vi "Intake Controller.vi"(8 "error in":errorcluster) -> ()   [LabVIEW 2017]
doc: "This VI executes continuously carrying out the current operation and responding to updates or new operations. It will often contain the timing or control code that is difficult to place directly in TeleOp. This VI generally opens all sensors and motors and isolates the rest of the robot code from knowing how the operations are carried out."
uses:
  Intake Operations.ctl
  Intake Setpoints.ctl
  <vilib>/Rock Robotics/WPI/SafetyOutput/WPI_SafetyOutputConfigMenu.ctl
  <vilib>/Rock Robotics/SystemInterfaces/DIO/FPGA_DIOPWMChannel.ctl
  <vilib>/Rock Robotics/WPI/RobotDrive/WPI_RobotDriveOpen2MotorWithSPARK.vi
  <vilib>/Rock Robotics/WPI/RobotDrive/WPI_RobotDriveOpen4MotorWithSPARK.vi
  <vilib>/Rock Robotics/Network Tables/NT Write Boolean.vi
  <vilib>/Rock Robotics/WPI/Solenoid/WPI_SolenoidOpenSingle.vi
  <vilib>/Rock Robotics/WPI/Solenoid/WPI_SolenoidChannel.ctl
  <vilib>/Rock Robotics/WPI/Framework/Completion Status.ctl
panel:
  in  "Interactive Values":T1
  out "Current\nCmd":string
  in  "Buttons":cluster{"Execute Cmd":bool, "Abort Cmd":bool}
  out "Command Timing":cluster{"Start Time (ms)":u32, "Iterations":i32}
  out "Status":T3
  # "Tip: It may be helpful to observe inputs and sensor values.\nYou may also want to display tuning or debugging controls."
  # "Interactive Command: You may fill in the settings for a command\nand schedule it with the Execute button. You can observe and abort\nany command while fine tuning the code for the controller."
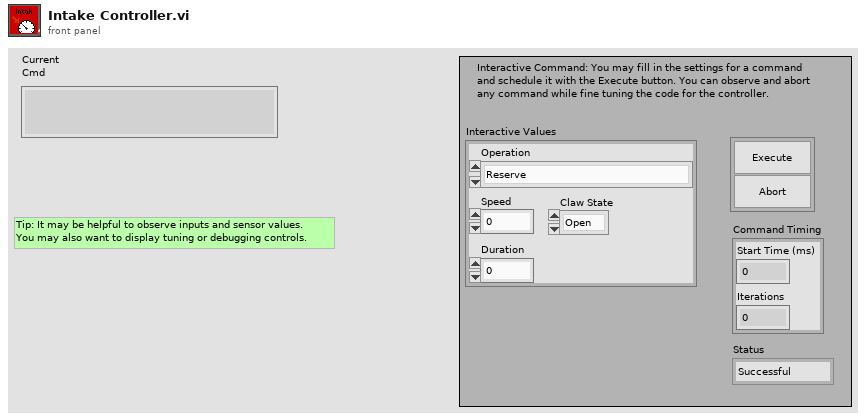
[diagram p1: front panel]
types:
  T1 = typedef "Intake Setpoints.ctl" = cluster{"Operation":T2, "Speed":dbl, "Duration":dbl, "Claw State":enum16{"Open", "Closed"}}
  T2 = typedef "Intake Operations.ctl" = enum16{"Reserve", "Read Current", "Immediate", "Open and Close Claw", "Intake for Duration", "Intake Until Cube"}
  T3 = typedef "Completion Status.ctl" = enum16{"Successful", "Aborted", "Incomplete"}
  T4 = typedef "WPI_SolenoidChannel.ctl" = enum8{"Solenoid 0", "Solenoid 1", "Solenoid 2", "Solenoid 3", "Solenoid 4", "Solenoid 5", "Solenoid 6", "Solenoid 7", "Invalid"}
  T5 = typedef "WPI_SafetyOutputConfigMenu.ctl" = enum16{"Enable", "Disable"}
  T6 = typedef "FPGA_DIOPWMChannel.ctl" = enum8{"PWM 0", "PWM 1", "PWM 2", "PWM 3", "PWM 4", "PWM 5", "PWM 6", "PWM 7", "PWM 8", "PWM 9", "PWM MXP 0", "PWM MXP 1", "PWM MXP 2", "PWM MXP 3", "PWM MXP 4", "PWM MXP 5", "PWM MXP 6", "PWM MXP 7", "PWM MXP 8", "PWM MXP 9", "Invalid"}
  T7 = typedef "WPI_RobotDriveDevRef.ctl" = cluster{"DevStatus":errorcluster, "Motors[]":T8[], "Square Inputs":bool, "Max Output":dbl}
  T8 = typedef "WPI_MotorControlDeviceRef.ctl" = cluster{"DeviceStatus":errorcluster, "Type":T9, "PWM":cluster{"PWM Channel":T6, "DeadBand":T10}, "CAN":cluster{"Device Number":u8, "SetOutput VI Ref":variant, "GetOutput VI Ref":variant, "Enable VI Ref":variant, "Disable VI Ref":variant, "Data":variant}, "Invert":bool, "DIO PWM":cluster{"PWM \"Enable\" Channel":T6, "DIOChannel":T11, "PWM Rate":dbl}}
  T9 = typedef "WPI_MotorControlType.ctl" = enum16{"PWM", "CAN", "DIO PWM"}
  T10 = typedef "WPI_PWMDeadband.ctl" = cluster{"Name":string, "maxPositivePwm":i32, "minPositivePwm":i32, "centerPwm":i32, "maxNegativePwm":i32, "minNegativePwm":i32, "angularRange":u16}
  T11 = typedef "FPGA_DIOChannel.ctl" = enum8{"DIO 0", "DIO 1", "DIO 2", "DIO 3", "DIO 4", "DIO 5", "DIO 6", "DIO 7", "DIO 8", "DIO 9", "DIO MXP 0", "DIO MXP 1", "DIO MXP 2", "DIO MXP 3", "DIO MXP 4", "DIO MXP 5", "DIO MXP 6", "DIO MXP 7", "DIO MXP 8", "DIO MXP 9", "DIO MXP 10", "DIO MXP 11", "DIO MXP 12", "DIO MXP 13", "DIO MXP 14", "DIO MXP 15", "SPI Port CS1", "SPI Port CS2", "SPI Port CS3", "SPI Port MISO", "SPI Port MOSI", "Invalid"}
  T12 = cluster{"RobotDriveDevRef":T7, "RobotDriveDevRef":T7}
  T13 = typedef "Command Status Info.ctl" = cluster{"Name":string, "Status":T3, "notifier out":T14}
  T14 = typedef "Completion Notifier.ctl" = refnum<notifier>
  T15 = cluster{"Current Command":T1, "Command Timing":cluster{"Start Time (ms)":u32, "Iterations":i32}, "Command Arguments":cluster{"Command Info":T13, "Description":string, "Default Command":T1, "queue out":refnum<queue>, "Subsystem Name":string}}
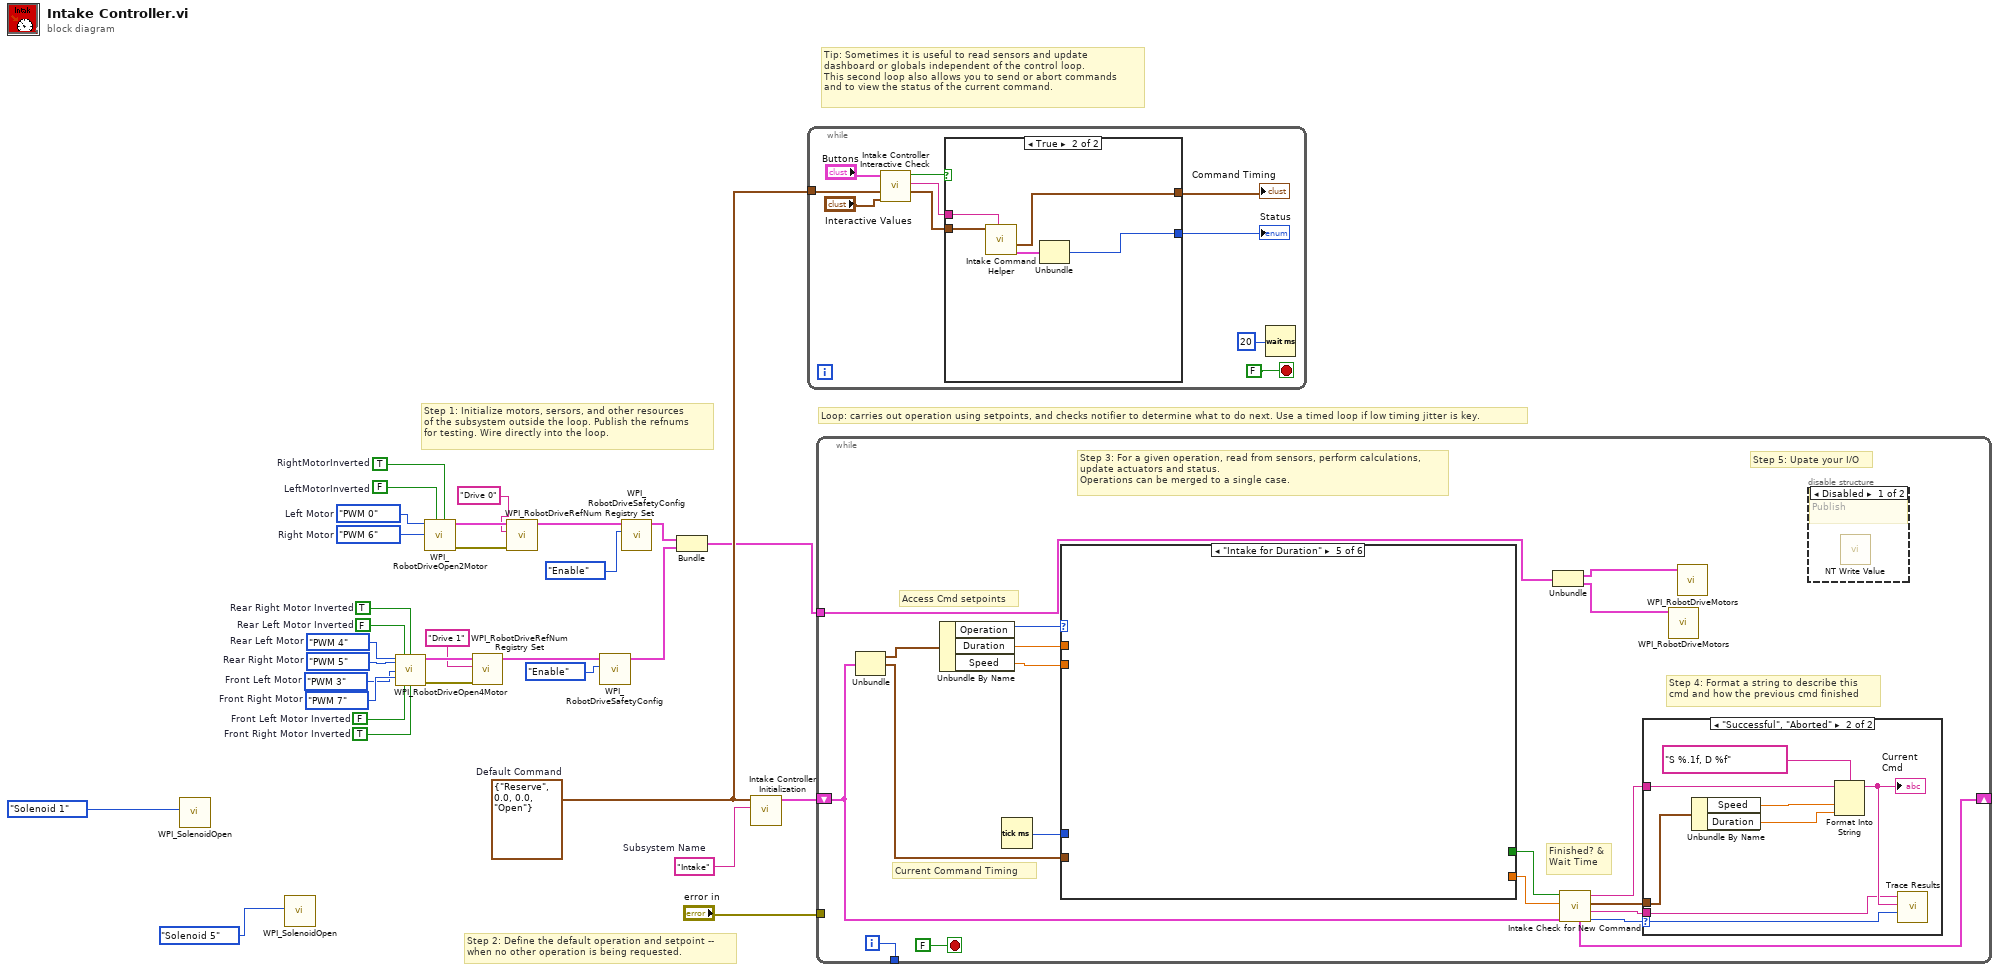
[diagram p0: block diagram]
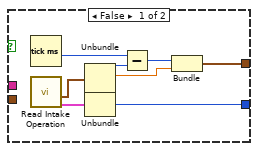
[diagram p2: hidden frame]
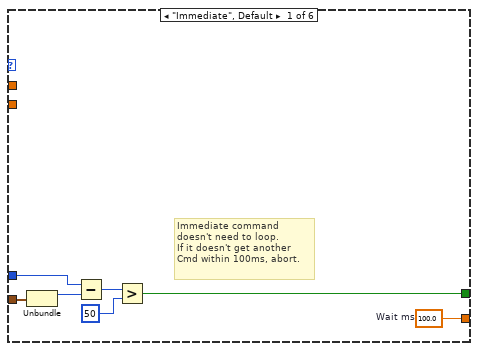
[diagram p5: hidden frame]
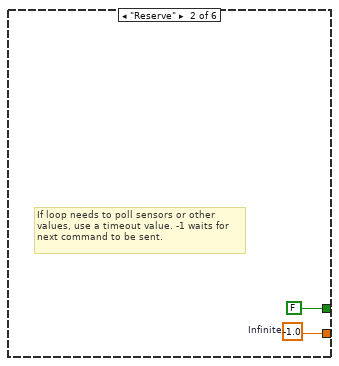
[diagram p6: hidden frame]
diagram:
  w6 = TRUE  # Front Right Motor Inverted
  w7 = FALSE  # Front Left Motor Inverted
  w8 = TRUE  # Rear Right Motor Inverted
  w9 = FPGA_DIOPWMChannel."PWM 4"  # Rear Left Motor
  w10 = FPGA_DIOPWMChannel."PWM 3"  # Front Left Motor
  w11 = FPGA_DIOPWMChannel."PWM 5"  # Rear Right Motor
  w12 = FALSE  # Rear Left Motor Inverted
  w13 = FPGA_DIOPWMChannel."PWM 7"  # Front Right Motor
  w19 = TRUE  # RightMotorInverted
  w20 = FPGA_DIOPWMChannel."PWM 6"  # Right Motor
  w21 = FPGA_DIOPWMChannel."PWM 0"  # Left Motor
  w22 = FALSE  # LeftMotorInverted
  w28 = T1 {"Operation"=enum."Reserve", "Speed"=0.0, "Duration"=0.0, "Claw State"=enum."Open"}  # Default Command
  w29 = "Intake"  # Subsystem Name
  # "Tip: Sometimes it is useful to read sensors and update\ndashboard or globals independent of the control loop.\nThis second loop also allows you to send or abort commands\nand to view the status of the current command."
  # "Step 2: Define the default operation and setpoint --\nwhen no other operation is being requested."
  # "Step 1: Initialize motors, sersors, and other resources\nof the subsystem outside the loop. Publish the refnums\nfor testing. Wire directly into the loop."
  # "Loop: carries out operation using setpoints, and checks notifier to determine what to do next. Use a timed loop if low timing jitter is key."
  n1 = call-poly <vilib>:"WPI_SolenoidOpen.vi"("Solenoid Channel"=WPI_SolenoidChannel."Solenoid 1") -> ()  [unwired: 9 in, 2 out]
  n2 = call-poly <vilib>:"WPI_SolenoidOpen.vi"("Solenoid Channel"=WPI_SolenoidChannel."Solenoid 5") -> ()  [unwired: 9 in, 2 out]
  n3 = call-poly <vilib>:"WPI_RobotDriveOpen4Motor.vi"("Rear Left Motor"=w9, "Rear Left Motor Inverted"=w12, "Rear Right Motor Inverted"=w8, "Rear Right Motor"=w11, "Front Left Motor"=w10, "Front Right Motor"=w13, "Front Left Motor Inverted"=w7, "Front Right Motor Inverted"=w6) -> ("RobotDriveDevRef"=w15:T7, "error out"=w14:errorcluster)  [unwired: 6 in]
  n4 = call-poly <vilib>:"WPI_RobotDriveOpen2Motor.vi"("Right Motor Inverted"=w19, "Left Motor Inverted"=w22, "Right Motor"=w20, "Left Motor"=w21) -> ("error out"=w24:errorcluster, "RobotDriveDevRef"=w23:T7)  [unwired: 1 in, 5 out]
  n5 = call <vilib>:"WPI_RobotDriveRefNum Registry Set.vi"("error in (no error)"=w14, "refnum name"="Drive 1", "RobotDriveDevRef"=w15) -> ("RobotDriveDevRef"=w16:T7)  [unwired: 1 in, 7 out]
  n6 = call <vilib>:"WPI_RobotDriveRefNum Registry Set.vi"("error in (no error)"=w24, "refnum name"="Drive 0", "RobotDriveDevRef"=w23) -> ("RobotDriveDevRef"=w25:T7)  [unwired: 1 in, 7 out]
  n7 = call <vilib>:"WPI_RobotDriveSafetyConfig.vi"("mode"=WPI_SafetyOutputConfigMenu."Enable", "RobotDriveDevRef"=w16) -> ("RobotDriveDevRef"=w17:T7)  [unwired: 8 in, 1 out]
  n8 = call <vilib>:"WPI_RobotDriveSafetyConfig.vi"("mode"=WPI_SafetyOutputConfigMenu."Enable", "RobotDriveDevRef"=w25) -> ("RobotDriveDevRef"=w26:T7)  [unwired: 8 in, 1 out]
  n9 = Bundle("RobotDriveDevRef"=w26, "RobotDriveDevRef"=w17) -> (w3:T12)  [unwired: 1 in]
  n10 = call "Intake Controller Initialization.vi"("Subsystem Name"=w29, "Default Command"=w28) -> ("Current Command"=w30:T15)  [unwired: 9 in]
  n11 = while {
    tunnel: w28 -> [w38]
    stop <- FALSE stop-if-true
    n12 = call "Intake Controller Interactive Check.vi"("Interactive Command in"="Interactive Values", "Default Command"=w38, "Buttons"="Buttons") -> ("Interactive Command out"=w35:T1, "Trace String"=w36:string, "Schedule"=w37:bool)  [unwired: 6 in]
    n13 = case shown="True" w37 {
      tunnel: [w49 w54] -> w34
      tunnel: w35 -> [_ w52]
      tunnel: [w45 w50] -> w33
      tunnel: w36 -> [_ w53]
      frame False {
        n14 = Tick Count (ms)() -> (millisecond timer value=w44:u32)
        n15 = call "Read Intake Operation.vi"() -> ("Command Info"=w42:T13, "SubSystem Data"=w43:T1)  [unwired: 9 in, 1 out]
        n16 = Unbundle(w43) -> ("Operation"=w48:T2, "Speed"=w46:dbl)  [unwired: 2 out]
        n17 = Unbundle(w42) -> ("Status"=w49:T3)  [unwired: 2 out]
        n18 = Subtract(x=w44, y=w48) -> (x-y=w47:u32)
        n19 = Bundle(w47, "Speed"=w46) -> (w45:cluster{u32, "Speed":dbl})  [unwired: 1 in]
      }
      frame True {
        n20 = call "Intake Command Helper.vi"("Description"=w53, "SubSystem Data"=w52) -> ("Command Info Out"=w51:T13, "Command Timing"=w50:cluster{"Start Time (ms)":u32, "Iterations":i32})  [unwired: 7 in, 1 out]
        n21 = Unbundle(w51) -> ("Status"=w54:T3)  [unwired: 2 out]
      }
    }
    "Status" <- w34
    "Command Timing" <- w33
    n22 = Wait (ms)(milliseconds to wait=u32 20) -> ()  [unwired: 1 out]
  }
  n23 = while {
    shift-right: [w65] -> _
    shift-left: w30 -> [w58]
    tunnel: [w72] -> _
    tunnel: "error in" -> [_]
    tunnel: w3 -> [w55]
    i -> [w72]
    stop <- FALSE stop-if-true
    # "Step 5: Upate your I/O"
    # "Step 4: Format a string to describe this\ncmd and how the previous cmd finished"
    # "Current Command Timing"
    # "Access Cmd setpoints"
    # "Finished? &\nWait Time"
    # "Step 3: For a given operation, read from sensors, perform calculations,\nupdate actuators and status.\nOperations can be merged to a single case."
    n24 = Unbundle(w58) -> ("Current Command"=w71:T1, "Command Timing"=w67:cluster{"Start Time (ms)":u32, "Iterations":i32})  [unwired: 1 out]
    n25 = Unbundle By Name(w71) -> ("Operation"=w70:T2, "Duration"=w69:dbl, "Speed"=w66:dbl)
    n26 = Tick Count (ms)() -> (millisecond timer value=w68:u32)
    n27 = case shown="\"Intake for Duration\"" w70 {
      tunnel: [w88 w90 _ _ _ _] -> w63
      tunnel: [w82 FALSE ("ignore previous (F)") _ _ _ _] -> w64
      tunnel: w67 -> [w84 _ _ _ _ _]
      tunnel: w69 -> [_ _ _ _ _ _]
      tunnel: w68 -> [w83 _ _ _ _ _]
      tunnel: w66 -> [_ _ _ _ _ _]
      frame "Immediate", Default {
        w88 = 100.0  # Wait ms
        # "Immediate command\ndoesn't need to loop.\nIf it doesn't get another\nCmd within 100ms, abort."
        n28 = Unbundle(w84) -> ("Start Time (ms)"=w87:u32)  [unwired: 1 out]
        n29 = Subtract(x=w83, y=w87) -> (x-y=w86:u32)
        n30 = Greater?(x=w86, y=u8 50 ("Left Motor")) -> (0:w82:bool)
      }
      frame "Reserve" {
        w90 = -1.0  # Infinite
        # "If loop needs to poll sensors or other\nvalues, use a timeout value. -1 waits for\nnext command to be sent."
      }
      frame "Read Current" {
      }
      frame "Open and Close Claw" {
      }
      frame "Intake for Duration" {
      }
      frame "Intake Until Cube" {
      }
    }
    n31 = Unbundle(w55) -> ("RobotDriveDevRef"=w56:T7, "RobotDriveDevRef"=w57:T7)
    n32 = call "Intake Check for New Command.vi"("Current Command"=w58, "Wait time (ms)"=w63, "Finished?"=w64) -> ("Completion"=w59:T3, "Subsystem Name"=w60:string, "Current Command"=w61:T1, "Initial Trace String"=w62:string, "NextCommand"=w65:T15)  [unwired: 4 in]
    n33 = case shown="\"Successful\", \"Aborted\"" w59 {
      selector: w59 -> [_ w81]
      tunnel: w62 -> [_ w77]
      tunnel: w61 -> [_ w78]
      tunnel: w60 -> [_ w74]
      frame "Incomplete", Default {
        # "Continuing current command"
      }
      frame "Successful", "Aborted" {
        # "Report and setup for next command"
        n34 = Unbundle By Name(w78) -> ("Speed"=w80:dbl, "Duration"=w75:dbl)
        n35 = Format Into String(format string="S %.1f, D %f", initial string=w77, w80, w75) -> (resulting string=w76:string)  [unwired: 1 in, 1 out]
        "Current\nCmd" <- w76
        n36 = call <vilib>:"Trace Results.vi"("Status of previous command"=w81, "Description"=w76, "Subsystem"=w74) -> ()  [unwired: 9 in]
      }
    }
    n37 = call <vilib>:"WPI_RobotDriveMotors.vi"("RobotDriveDevRef"=w57) -> ()  [unwired: 3 in, 8 out]
    n38 = call <vilib>:"WPI_RobotDriveMotors.vi"("RobotDriveDevRef"=w56) -> ()  [unwired: 3 in, 8 out]
    n39 = disable-structure shown="Disabled" {
      frame Disabled {
        # "Publish"
        n40 = call-poly <vilib>:"NT Write Value.vi"() -> ()  [unwired: 11 in, 1 out]
      }
      frame Enabled {
      }
    }
  }
